vi "messageClient.vi"() -> ()   [LabVIEW 2015]
panel:
  out "error out":errorcluster
  in  "queueName":string="messageQue"
  in  "OK Button":bool
  in  "port":u16
  in  "ip":string="127.0.0.1"
  out "MessageLog":string[](array[string])
  in  "data in":string="0002ab"
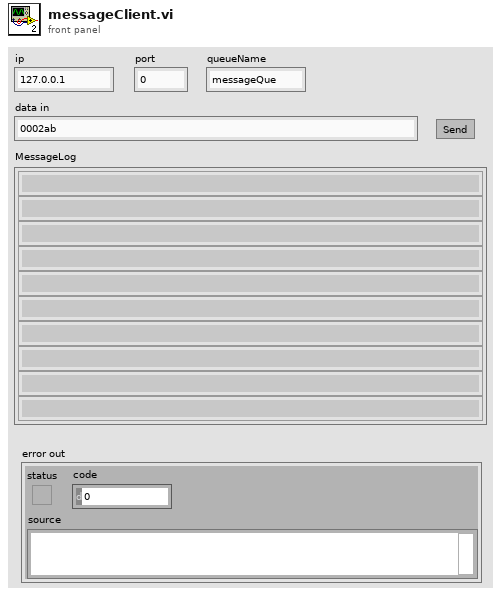
[diagram p1: front panel]
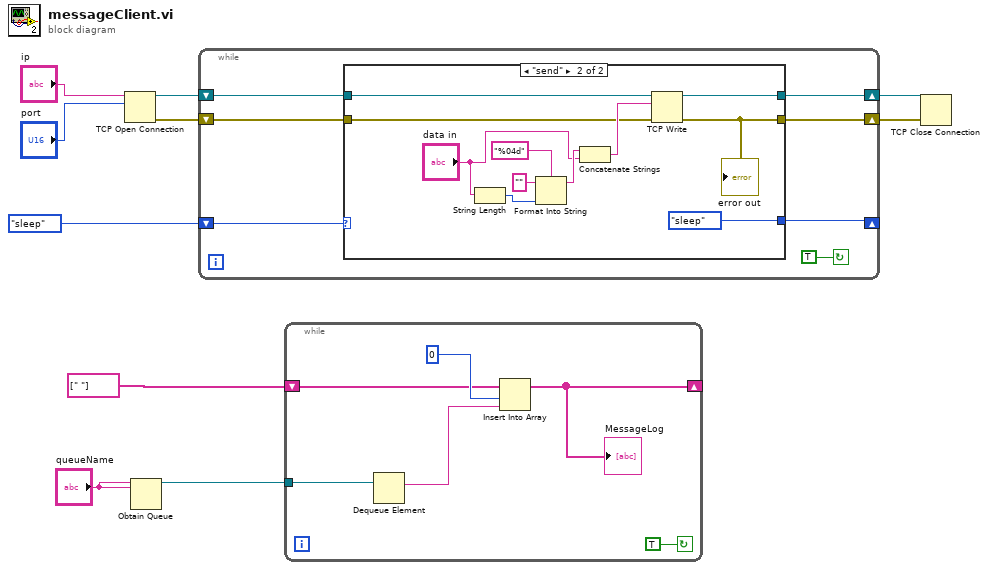
[diagram p0: block diagram]
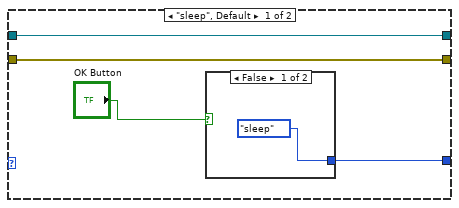
[diagram p2: hidden frame]
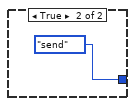
[diagram p3: hidden frame]
diagram:
  n1 = TCP Open Connection(address="ip", remote port or service name="port") -> (connection ID=w4:refnum<k5>, error out=w3:errorcluster)  [unwired: 3 in]
  n2 = Obtain Queue(name (unnamed)="queueName", element data type="queueName") -> (queue out=w9:refnum<queue>)  [unwired: 3 in, 2 out]
  n3 = while {
    shift-right: [w15] -> _
    shift-left: enum16{"sleep", "send"}."sleep" ("Enum") -> [w16]
    shift-right: [w13] -> w2
    shift-left: w4 -> [w14]
    shift-right: [w11] -> w1
    shift-left: w3 -> [w12]
    stop <- TRUE continue-if-true
    n4 = case shown="\"send\"" w16 {
      tunnel: [w20 enum16{"sleep", "send"}."sleep" ("Enum")] -> w15
      tunnel: w14 -> [w19 w27]
      tunnel: [w19 w26] -> w13
      tunnel: w12 -> [w18 w25]
      tunnel: [w18 w24] -> w11
      frame "sleep", Default {
        n5 = case shown="False" "OK Button" {
          tunnel: [enum16{"sleep", "send"}."sleep" ("Enum") enum16{"sleep", "send"}."send" ("Enum")] -> w20
          frame False {
          }
          frame True {
          }
        }
      }
      frame "send" {
        n6 = String Length(string="data in") -> (length=w34:i32)
        n7 = Format Into String(format string="%04d", initial string="", w34) -> (resulting string=w32:string)  [unwired: 1 in, 1 out]
        n8 = Concatenate Strings(w32, "data in") -> (w30:string)
        n9 = TCP Write(connection ID=w27, data in=w30, error in (no error)=w25) -> (connection ID out=w26:refnum<k5>, error out=w24:errorcluster)  [unwired: 1 in, 1 out]
        "error out" <- w24
      }
    }
  }
  n10 = while {
    tunnel: w9 -> [w40]
    shift-right: [w35] -> _
    shift-left: string[] [" "] ("Array") -> [w37]
    stop <- TRUE continue-if-true
    n11 = Dequeue Element(queue=w40) -> (element=w38:string)  [unwired: 2 in, 3 out]
    n12 = Insert Into Array(array=w37, index=0, new element=w38) -> (w35:string[])
    "MessageLog" <- w35
  }
  n13 = TCP Close Connection(connection ID=w2, error in (no error)=w1) -> ()  [unwired: 1 in, 2 out]
